vi "BindingVI.vi"(6 "Library Path":path, 8 "error in":errorcluster, 11 "Binding info":string[][](array[string])) -> (0 "error out":errorcluster, 2 "Error status":bool)   [LabVIEW 2014]
doc: "<B>Copyright</B>: (c) 2015 MHWirth. All rights reserved.\n\nThis subVI binds every shared variable in the library to the specified shared variable. It requires a 2D Array of strings. The first column is the names, the 3rd, 4th, and 5th are the server name, the process name, and the variable name of the binding variable. The 2nd column, which is data type, is not in use."
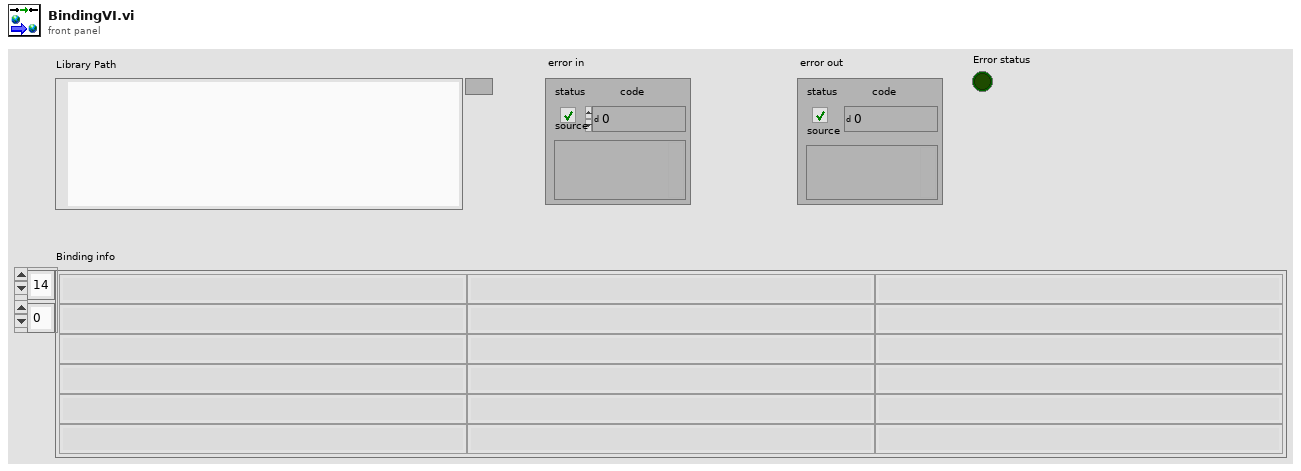
[diagram p1: front panel]
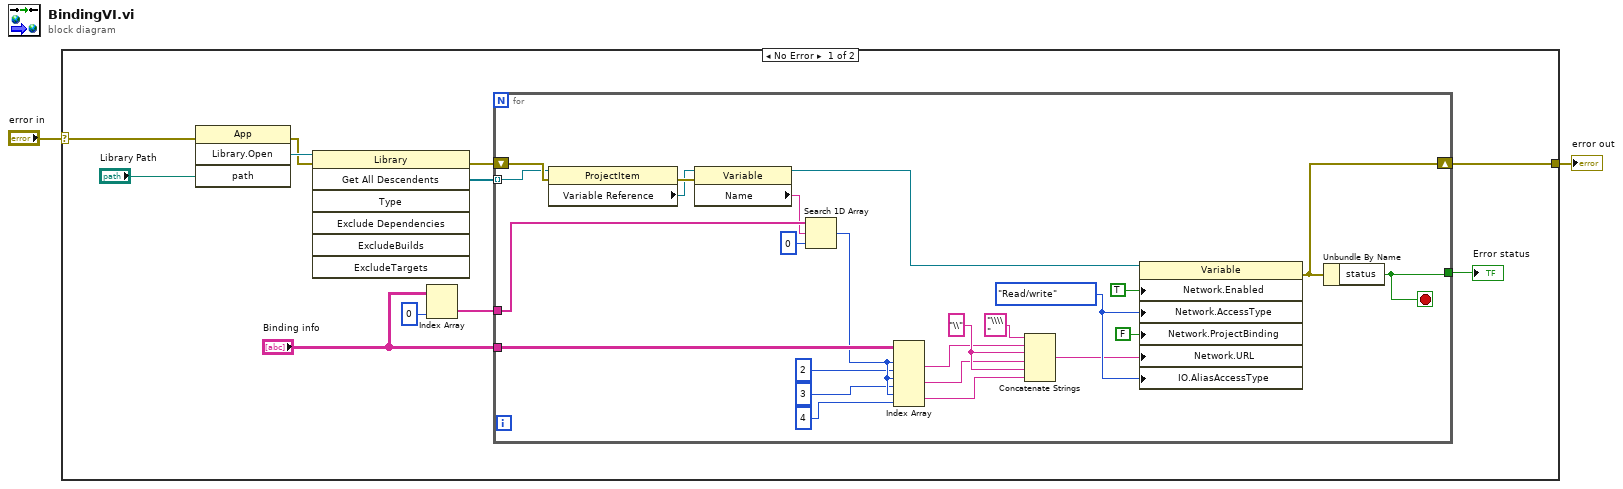
[diagram p0: block diagram]
diagram:
  n1 = case shown="No Error" "error in" {
    selector: "error in" -> [w10 w38]
    tunnel: [w7 w38] -> w1
    frame No Error {
      n2 = invoke class="App" method="Library.Open"(error in=w10, "path"="Library Path") -> (error out=w9:errorcluster, "Open Library"=w12:refnum<vi>)  [unwired: 2 in, 2 out]
      n3 = invoke class="Library" method="Get All Descendents"(reference=w12, error in=w9) -> (error out=w8:errorcluster, "All Descendents"=w11:refnum<vi>[])  [unwired: 5 in, 5 out]
      n4 = Index Array(array="Binding info", index (col)=0 ("disabled index (col)")) -> (element=w3:string[])  [unwired: 1 in]
      n5 = for {
        tunnel: w11 -> [w25] mode=indexing
        shift-right: [w31] -> w7
        shift-left: w8 -> [w26]
        tunnel: [w30] -> w6
        tunnel: "Binding info" -> [w19]
        tunnel: w3 -> [w22]
        stop <- w30 stop-if-true
        w33 = "\\" ("string")
        w35 = enum32{"Read only", "Write only", "Read/write"}."Read/write" ("Network:Access Type")
        n6 = property class="ProjectItem"(reference=w25, error in=w26) -> (error out=w24:errorcluster, "Variable Reference"=w23:refnum<vi>)  [unwired: 1 out]
        n7 = property class="Variable"(reference=w23, error in=w24) -> (reference out=w14:refnum<vi>, "Name"=w21:string)  [unwired: 1 out]
        n8 = Search 1D Array(1D array=w22, element=w21, start index (0)=0) -> (index of element=w18:i32)
        n9 = Index Array(array=w19, index (row) #1=w18, index (col) #1=2 ("disabled index (col)"), index (row) #2=w18, index (col) #2=3 ("disabled index (col)"), index (row) #3=w18, index (col) #3=4 ("disabled index (col)")) -> (element #1=w29:string, element #2=w28:string, element #3=w27:string)
        n10 = Concatenate Strings("\\\\" ("string"), w29, w33, w28, w33, w27) -> (w32:string)
        n11 = property class="Variable"(reference=w14, "Network.Enabled"=TRUE ("Network:Use Binding"), "Network.AccessType"=w35, "Network.ProjectBinding"=FALSE ("Network:Project Binding"), "Network.URL"=w32, "IO.AliasAccessType"=w35) -> (error out=w31:errorcluster)  [unwired: 1 in, 1 out]
        n12 = Unbundle By Name(w31) -> ("status"=w30:bool)
      }
      "Error status" <- w6
    }
    frame Error {
    }
  }
  "error out" <- w1
